vi "New.vi"(0 "RFFE Command in":refnum<class "RFFE Command.lvclass">, 1 "Alias":string, 5 "Slave Address":T2=12 format="%02x", 7 "Register Address":T1 format="%02x", 11 "error in (no error)":errorcluster) -> (4 "RFFE Command out":refnum<class "RFFE Command.lvclass">, 15 "error out":errorcluster)   [LabVIEW 2018, in "MIPI RFFE API.lvlib" / "RFFE Command.lvclass"]
uses:
  RFFE Command.lvclass
  Slave Address.ctl
  Register Address.ctl
  RFFE Command.lvclass/RFFE Command.ctl
  MIPI RFFE API.lvlib
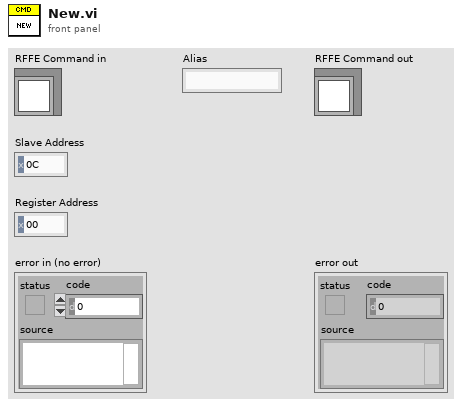
[diagram p1: front panel]
types:
  T1 = typedef "MIPI RFFE API.lvlib/Register Address.ctl" = u16
  T2 = typedef "MIPI RFFE API.lvlib/Slave Address.ctl" = u8
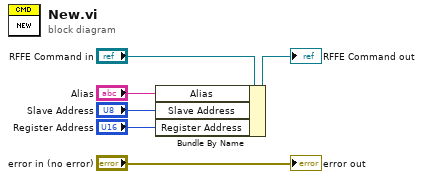
[diagram p0: block diagram]
diagram:
  n1 = Bundle By Name(cluster="RFFE Command in", "Alias"="Alias", "Slave Address"="Slave Address", "Register Address"="Register Address") -> (→"RFFE Command out":refnum<class "RFFE Command.lvclass">)
  "error out" <- "error in (no error)"
